vi "CAN process.vi"(4 "error in (no error)":errorcluster, 5 "Data":u8[](array[numeric]), 6 "COB id":i32, 7 "CANopen in":refnum<class "CANopen.lvclass">) -> (0 "error out":errorcluster, 2 "Processed?":bool, 3 "CANopen out":refnum<class "CANopen.lvclass">)   [LabVIEW 2024, in "canopen.lvlib" / "CANopen.lvclass"]
doc: "Tries to store the data of a COB (usually a PDO message) into the input image. The correct COB-ID must be previously set in the input map, that is usually registered with \"Set input map\" prior to this call. \"\"Processed?\" is set to true if the given message matches an entry on the map, in which case data is put inside its reserved space in the internally owned input image."
uses:
  CANopen.lvclass
  CANopen.lvclass/CANopen.ctl
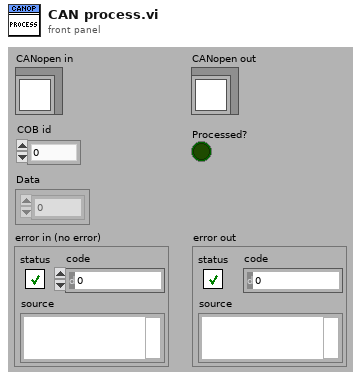
[diagram p1: front panel]
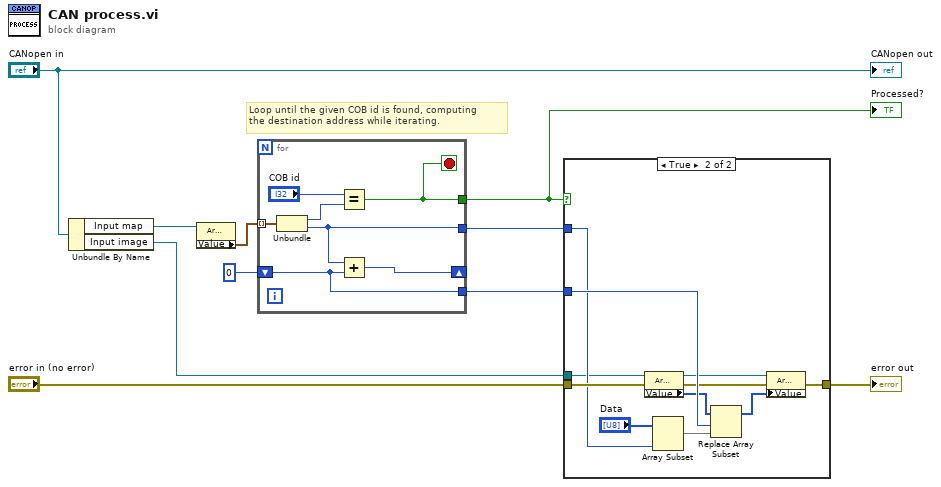
[diagram p0: block diagram]
diagram:
  # "Loop until the given COB id is found, computing\nthe destination address while iterating."
  n1 = Unbundle By Name("CANopen in") -> ("Input map"=w3:refnum<vi>, "Input image"=w2:refnum<vi>)
  n2 = property class="Arr (strict)"(reference=w3) -> ("Value"=w4:cluster{"CobID":u32, "nBytes":u8}[])  [unwired: 1 in, 2 out]
  n3 = for {
    tunnel: w4 -> [w17] mode=indexing
    shift-right: [w15] -> _
    shift-left: 0 -> [w14]
    tunnel: [w14] -> w8
    tunnel: [w13] -> w9
    tunnel: [w12] -> w7
    stop <- w13 stop-if-true
    n4 = Unbundle(w17) -> ("CobID"=w16:u32, "nBytes"=w12:u8)
    n5 = Equal?(x="COB id", y=w16) -> (x = y?=w13:bool)
    n6 = Add(x=w12, y=w14) -> (x+y=w15:i32)
  }
  "Processed?" <- w9
  n7 = case shown="True" w9 {
    tunnel: w8 -> [_ w28]
    tunnel: w7 -> [_ w20]
    tunnel: [w18 w22] -> w5
    tunnel: "error in (no error)" -> [w18 w21]
    tunnel: w2 -> [_ w19]
    frame False {
    }
    frame True {
      n8 = property class="Arr (strict)"(reference=w19, error in=w21) -> (reference out=w24:refnum<vi>, error out=w23:errorcluster, "Value"=w26:u8[])
      n9 = Array Subset(array="Data", length=w20) -> (w27:u8[])  [unwired: 1 in]
      n10 = Replace Array Subset(array=w26, new element=w27, index=w28) -> (w25:u8[])
      n11 = property class="Arr (strict)"(reference=w24, error in=w23, "Value"=w25) -> (error out=w22:errorcluster)  [unwired: 1 out]
    }
  }
  "error out" <- w5
  "CANopen out" <- "CANopen in"
